vi "Example Continuous.vi"() -> ()   [LabVIEW 2017]
uses:
  OS Simulator.lvlib
panel:
  in  "stop":bool
  out "Waveform Graph":waveform(dbl)(graph)
  in  "VISA resource name":refnum<visa-resource-name>="TCPIP::localhost::9996::SOCKET"
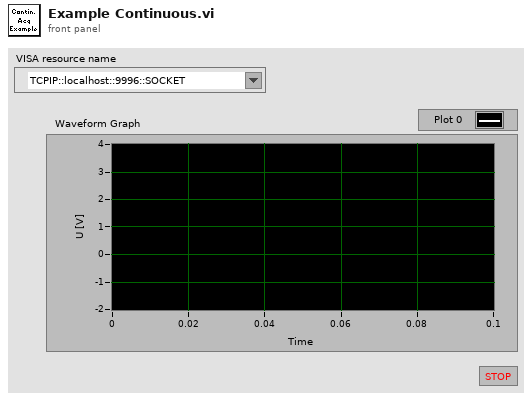
[diagram p1: front panel]
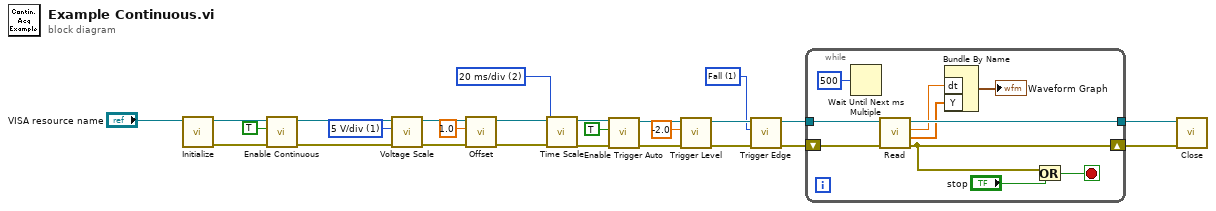
[diagram p0: block diagram]
diagram:
  w6 = u16 1 items=["Rise", "Fall"] ("Shape")
  w15 = u16 2 items=["200 ms/div", "100 ms/div", "20 ms/div"] ("Range")
  w21 = u16 1 items=["10 V/div", "5 V/div", "2 V/div", "1 V/div", "0.5 V/div", "0.1 V/div"] ("Range")
  n1 = call "Initialize.vi"("VISA resource name"="VISA resource name") -> ("error out"=w25:errorcluster, "VISA resource name out"=w26:refnum<visa-resource-name>)  [unwired: 9 in]
  n2 = call "Enable Continuous.vi"("error in (no error)"=w25, "Continous (Off)"=TRUE, "VISA resource name"=w26) -> ("error out"=w22:errorcluster, "VISA resource name out"=w23:refnum<visa-resource-name>)  [unwired: 7 in]
  n3 = call "Voltage Scale.vi"("error in"=w22, "Range"=w21, "VISA resource name"=w23) -> ("error out"=w19:errorcluster, "VISA resource name out"=w20:refnum<visa-resource-name>)  [unwired: 7 in]
  n4 = call "Offset.vi"("error in (no error)"=w19, "Offset (0)"=1.0, "VISA resource name"=w20) -> ("error out"=w17:errorcluster, "VISA resource name out"=w16:refnum<visa-resource-name>)  [unwired: 7 in]
  n5 = call "Time Scale.vi"("error in"=w17, "Range"=w15, "VISA resource name"=w16) -> ("error out"=w13:errorcluster, "VISA resource name out"=w14:refnum<visa-resource-name>)  [unwired: 7 in]
  n6 = call "Enable Trigger Auto.vi"("error in (no error)"=w13, "Enable (Off)"=TRUE, "VISA resource name"=w14) -> ("error out"=w10:errorcluster, "VISA resource name out"=w11:refnum<visa-resource-name>)  [unwired: 7 in]
  n7 = call "Trigger Level.vi"("error in (no error)"=w10, "Level (0)"=-2.0, "VISA resource name"=w11) -> ("error out"=w7:errorcluster, "VISA resource name out"=w8:refnum<visa-resource-name>)  [unwired: 7 in]
  n8 = call "Trigger Edge.vi"("error in (no error)"=w7, "Shape"=w6, "VISA resource name"=w8) -> ("error out"=w1:errorcluster, "VISA resource name out"=w4:refnum<visa-resource-name>)  [unwired: 7 in]
  n9 = while {
    tunnel: w4 -> [w36]
    tunnel: [w35] -> w3
    shift-right: [w30] -> w2
    shift-left: w1 -> [w34]
    stop <- w29 stop-if-true
    n10 = Wait Until Next ms Multiple(millisecond multiple=u32 500) -> ()  [unwired: 1 out]
    n11 = call "Read.vi"("error in"=w34, "VISA resource name"=w36) -> ("error out"=w30:errorcluster, "U [V]"=w32:dbl[], "dt [s]"=w33:dbl, "VISA resource name out"=w35:refnum<visa-resource-name>)  [unwired: 5 in, 1 out]
    n12 = Bundle By Name("dt"=w33, "Y"=w32) -> (→"Waveform Graph":waveform(dbl))  [unwired: 1 in]
    n13 = Or(x=w30, y="stop") -> (x .or. y?=w29:bool)
  }
  n14 = call "Close.vi"("error in (no error)"=w2, "VISA resource name"=w3) -> ()  [unwired: 9 in, 1 out]
